vi "Multiplier2.vi"() -> (8 "Multiplier2":refnum<class "Multiplier2.lvclass">)   [LabVIEW 2017, in "Multiplier2.lvclass"]
uses:
  Multiplier2.lvclass
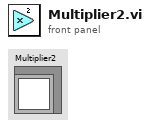
[diagram p1: front panel]
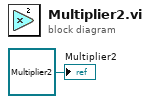
[diagram p0: block diagram]
diagram:
  "Multiplier2" <- refnum<class "Multiplier2.lvclass"> refnum ("Multiplier2.lvclass")
